vi "create_tracklogfile_header.vi"(1 "DEC":dbl format="%<%H:%M:%S%0u>t", 2 "H.A.":dbl format="%<%H:%M:%S%0u>t") -> (0 "Formatted header":string)   [LabVIEW 2011]
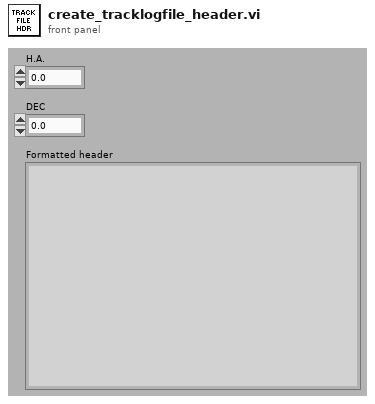
[diagram p1: front panel]
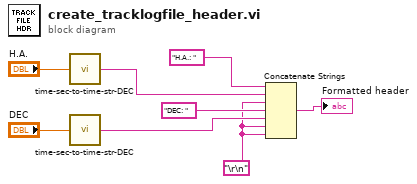
[diagram p0: block diagram]
diagram:
  w1 = "\r\n"
  n1 = call "time-sec-to-time-str-DEC.vi"("Numeric"="H.A.") -> ("formatted-str"=w5:string)
  n2 = call "time-sec-to-time-str-DEC.vi"("Numeric"="DEC") -> ("formatted-str"=w3:string)
  n3 = Concatenate Strings("H.A.: ", w5, w1, "DEC: ", w3, w1, w1) -> (→"Formatted header":string)
